vi "SPI PIXY Write Handler.vi"(8 "index":i32, 11 "Write Buffer":u8[](array[numeric])) -> (0 "SPI to Send":u8[](array[numeric]), 3 "Write Buffer out":u8[](array[numeric]))   [LabVIEW 2016]
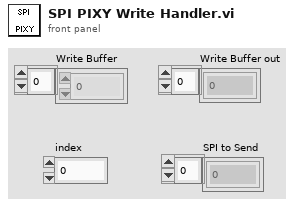
[diagram p1: front panel]
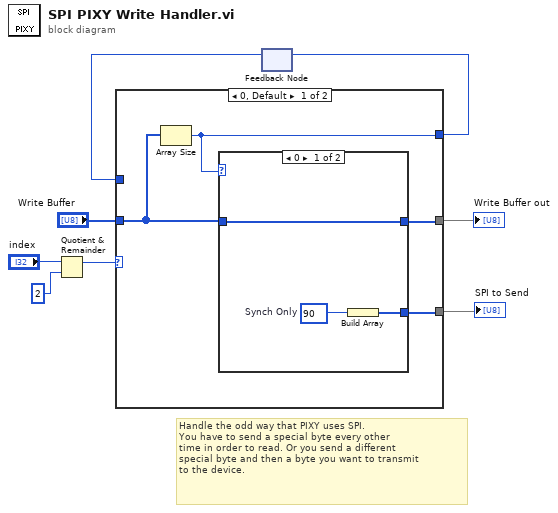
[diagram p0: block diagram]
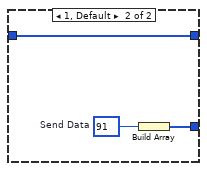
[diagram p2: hidden frame]
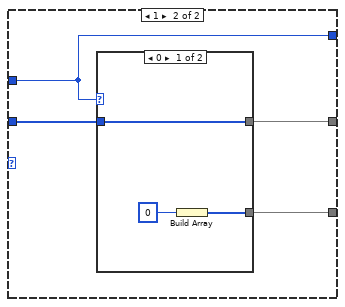
[diagram p3: hidden frame]
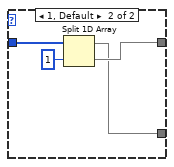
[diagram p4: hidden frame]
diagram:
  # "Handle the odd way that PIXY uses SPI.\nYou have to send a special byte every other\ntime in order to read. Or you send a different\nspecial byte and then a byte you want to transmit\nto the device."
  n1 = Quotient & Remainder(x="index", y=2) -> (x-y*floor(x/y)=w3:i32)  [unwired: 1 out]
  n2 = feedback #1() -> (w1:i32)  [unwired: 1 in]
  n3 = case shown="0, Default" w3 {
    tunnel: "Write Buffer" -> [w11 w22]
    tunnel: [w12 w21] -> w7
    tunnel: [w10 w20] -> w6
    tunnel: [w9 w19] -> w2
    tunnel: w1 -> [_ w19]
    frame 0, Default {
      n4 = Array Size(array=w11) -> (size(s)=w9:i32)
      n5 = case shown="0" w9 {
        tunnel: [w15 w16] -> w12
        tunnel: w11 -> [w15 w16]
        tunnel: [w13 w17] -> w10
        frame 0 {
          w14 = u8 90  # Synch Only
          n6 = Build Array(w14) -> (w13:u8[])
        }
        frame 1, Default {
          w18 = u8 91  # Send Data
          n7 = Build Array(w18) -> (w17:u8[])
        }
      }
    }
    frame 1 {
      n8 = case shown="0" w19 {
        tunnel: [w25 w28] -> w21
        tunnel: w22 -> [w25 w29]
        tunnel: [w24 w26] -> w20
        frame 0 {
          n9 = Build Array(u8 0) -> (w24:u8[])
        }
        frame 1, Default {
          n10 = Split 1D Array(array=w29, index=1) -> (first subarray=w26:u8[], second subarray=w28:u8[])
        }
      }
    }
  }
  "Write Buffer out" <- w7
  "SPI to Send" <- w6
  n11 = feedback-in #1(w2) -> ()
